vi "Use Mask Image File.vi"() -> ()   [LabVIEW 2011]
uses:
  <vilib>/picture/picture.llb/imagedata.ctl
panel:
  in  "Mask Color (Black)":u32(colorbox) caption="屏蔽颜色（黑色）"
  out "Mask Picture":picture
  out "picture":picture caption="Picture"
  out "Masked picture":picture caption="Masked Picture"
  in  "image data":T1={"image type"=0, "image depth"=24, "image"=array[49050 elements], "mask"=[], "colors"=[], "Rectangle"={"left"=0, "top"=0, "right"=109, "bottom"=150}} caption="图像数据"
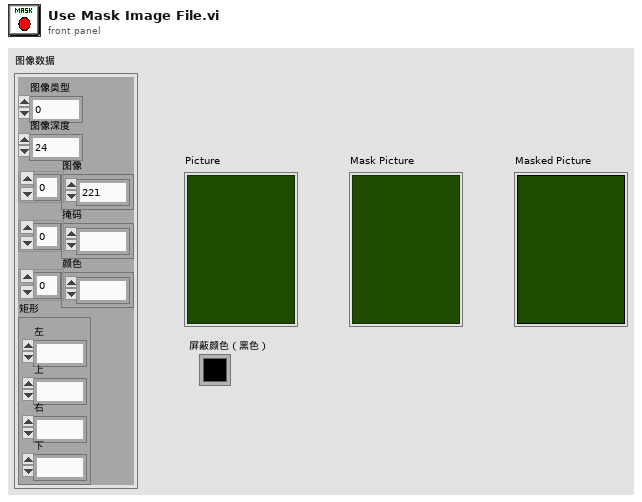
[diagram p1: front panel]
types:
  T1 = typedef "imagedata.ctl" = cluster{"image type":i32, "image depth":i32, "image":u8[], "mask":u8[], "colors":u32[], "Rectangle":cluster{"left":i16, "top":i16, "right":i16, "bottom":i16}}
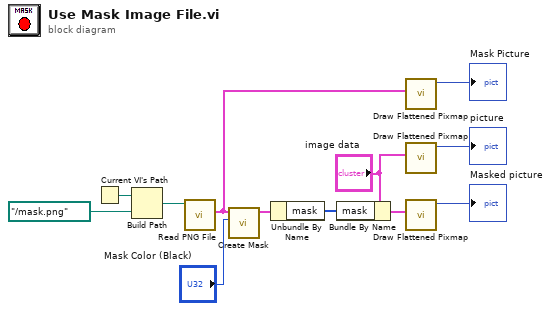
[diagram p0: block diagram]
diagram:
  n1 = Current VI's Path() -> (path=w4:path)
  n2 = Build Path(base path=w4, name or relative path=path "../mask.png") -> (appended path=w3:path)
  n3 = call <vilib>:"Read PNG File.vi"("path to PNG file"=w3) -> ("image data"=w2:T1)  [unwired: 8 in, 2 out]
  n4 = call <vilib>:"Create Mask.vi"("Mask Color (Black)"="Mask Color (Black)", "image data"=w2) -> ("image data"=w12:T1)  [unwired: 9 in]
  n5 = Unbundle By Name(w12) -> ("mask"=w11:u8[])
  n6 = Bundle By Name(cluster="image data", "mask"=w11) -> (w10:T1)
  n7 = call <vilib>:"Draw Flattened Pixmap.vi"("image data"=w2) -> ("new picture"=→"Mask Picture":picture)  [unwired: 8 in]
  n8 = call <vilib>:"Draw Flattened Pixmap.vi"("image data"="image data") -> ("new picture"=→"picture":picture)  [unwired: 8 in]
  n9 = call <vilib>:"Draw Flattened Pixmap.vi"("image data"=w10) -> ("new picture"=→"Masked picture":picture)  [unwired: 8 in]
